vi "ExSubCloseImage.vi"(1 "error in (no error)":errorcluster, 2 "Handles In":T1) -> (0 "error out":errorcluster)   [LabVIEW 2010]
panel:
  # "ExSubCloseImage:\nThis is a subVI which takes a cluster of handles and closes the and image only"
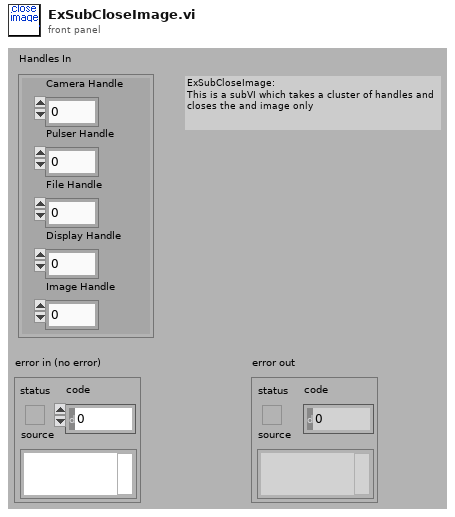
[diagram p1: front panel]
types:
  T1 = cluster{"Camera Handle":u32, "Pulser Handle":u32, "File Handle":u32, "Display Handle":u32, "Image Handle":u32}
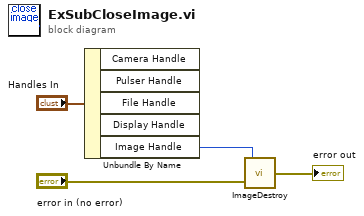
[diagram p0: block diagram]
diagram:
  n1 = Unbundle By Name("Handles In") -> ("Image Handle"=w3:u32)  [unwired: 4 out]
  n2 = call <userlib>:"ImageDestroy.vi"("error in"="error in (no error)", "Data handle"=w3) -> ("error out"=→"error out":errorcluster)
